vi "Get Number DDG External Outputs.vi"(8 "error in (no error)":errorcluster, 11 "puiCount":u32) -> (0 "error out":errorcluster, 2 "function return":u32, 3 "puiCount out":u32)   [LabVIEW 2014, in "atmcd32d.lvlib"]
doc: "unsigned int WINAPI GetNumberDDGExternalOutputs(at_u32 * puiCount);"
uses:
  atmcd32d.lvlib
  atmcd32d.dll
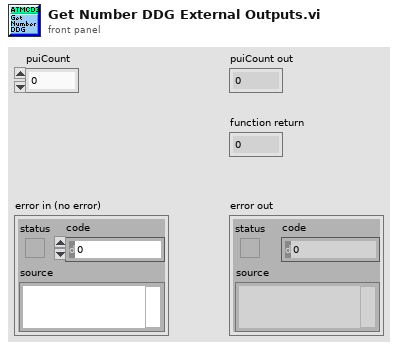
[diagram p1: front panel]
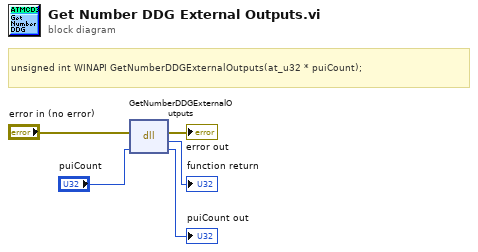
[diagram p0: block diagram]
diagram:
  # "unsigned int WINAPI GetNumberDDGExternalOutputs(at_u32 * puiCount);"
  n1 = dll-call lib="C:/Users/Bakir/Documents/Lambda2-Testing/lib/Andorlib/atmcd32d.*" fn="GetNumberDDGExternalOutputs"(error in="error in (no error)", "puiCount"="puiCount") -> (error out=→"error out":errorcluster, →"function return":u32, "puiCount"=→"puiCount out":u32)  [unwired: 2 in, 1 out]
